vi "fill cell loop.vi"(7 "Column Letter":string, 8 "error in (no error)":errorcluster, 9 "Row":i32, 10 "String":string, 11 "NI_report in":refnum<class "NI_report.lvclass">) -> (0 "error out":errorcluster, 3 "NI_report out":refnum<class "NI_report.lvclass">)   [LabVIEW 2016]
uses:
  <vilib>/Utility/NIReport.llb/NI_report.lvclass
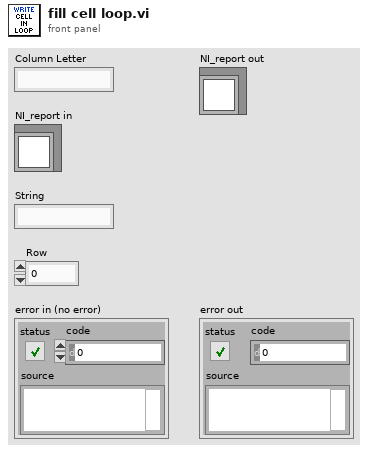
[diagram p1: front panel]
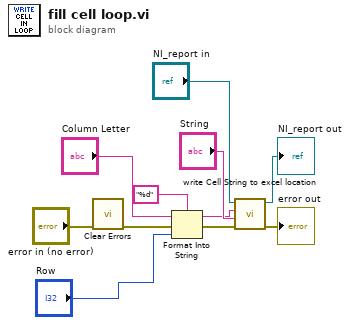
[diagram p0: block diagram]
diagram:
  n1 = call <vilib>:"Clear Errors.vi"("error in (no error)"="error in (no error)") -> ("error out"=w1:errorcluster)  [unwired: 5 in, 1 out]
  n2 = Format Into String(format string="%d", initial string="Column Letter", error in=w1, "Row") -> (resulting string=w5:string, error out=w4:errorcluster)
  n3 = call "write Cell String to excel location.vi"("error in (no error)"=w4, "input string"="String", "cell's name"=w5, "NI_report in"="NI_report in") -> ("error out"=→"error out":errorcluster, "NI_report out"=→"NI_report out":refnum<class "NI_report.lvclass">)  [unwired: 6 in]
